vi "SET_Origin.vi"(8 "error in":errorcluster, 10 "Point32":T1, 11 "Layer.lvclass in":refnum<class "Layer.lvclass">) -> (0 "error out":errorcluster, 3 "Layer.lvclass out":refnum<class "Layer.lvclass">)   [LabVIEW 2020, in "Layer.lvclass"]
doc: "Specify the Origin of the User Layer."
uses:
  Layer.lvclass
  Layer.lvclass/Layer.ctl
  <vilib>/Utility/miscctls.llb/LVPoint32TypeDef.ctl
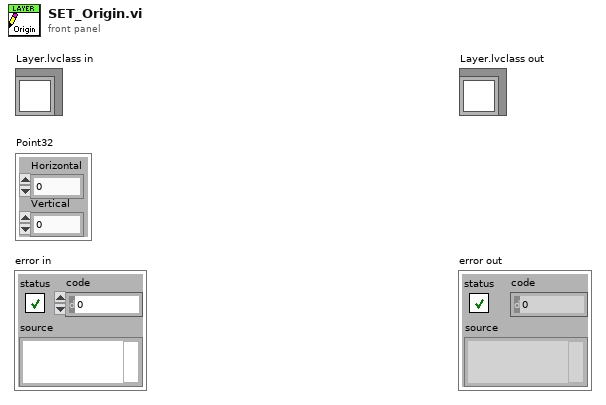
[diagram p1: front panel]
types:
  T1 = typedef "LVPoint32TypeDef.ctl" = cluster{"Horizontal":i32, "Vertical":i32}
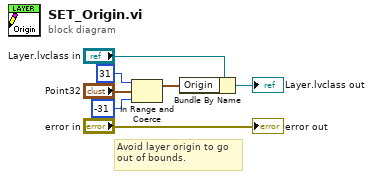
[diagram p0: block diagram]
diagram:
  # "Avoid layer origin to go\nout of bounds."
  n1 = In Range and Coerce(upper limit=31, x="Point32", lower limit=-31) -> (coerced(x)=w1:T1)  [unwired: 1 out]
  n2 = Bundle By Name(cluster="Layer.lvclass in", "Origin"=w1) -> (→"Layer.lvclass out":refnum<class "Layer.lvclass">)
  "error out" <- "error in"
